vi "Read_capp.vi"(7 "DELAY":u32, 8 "error in (no error)":errorcluster, 9 "String":string, 10 "REFF":refnum<visa-resource-name>, 11 "E4990A":refnum<visa-resource-name>) -> (0 "error out":errorcluster, 1 "Read Buffer":string, 2 "REFFout":refnum<visa-resource-name>, 3 "E4990A out":refnum<visa-resource-name>, 4 "data":dbl)   [LabVIEW 2012]
uses:
  <vilib>/Analysis/baseanly.llb/Mean (DBL).vi
  <vilib>/Analysis/NI_AALBase.lvlib
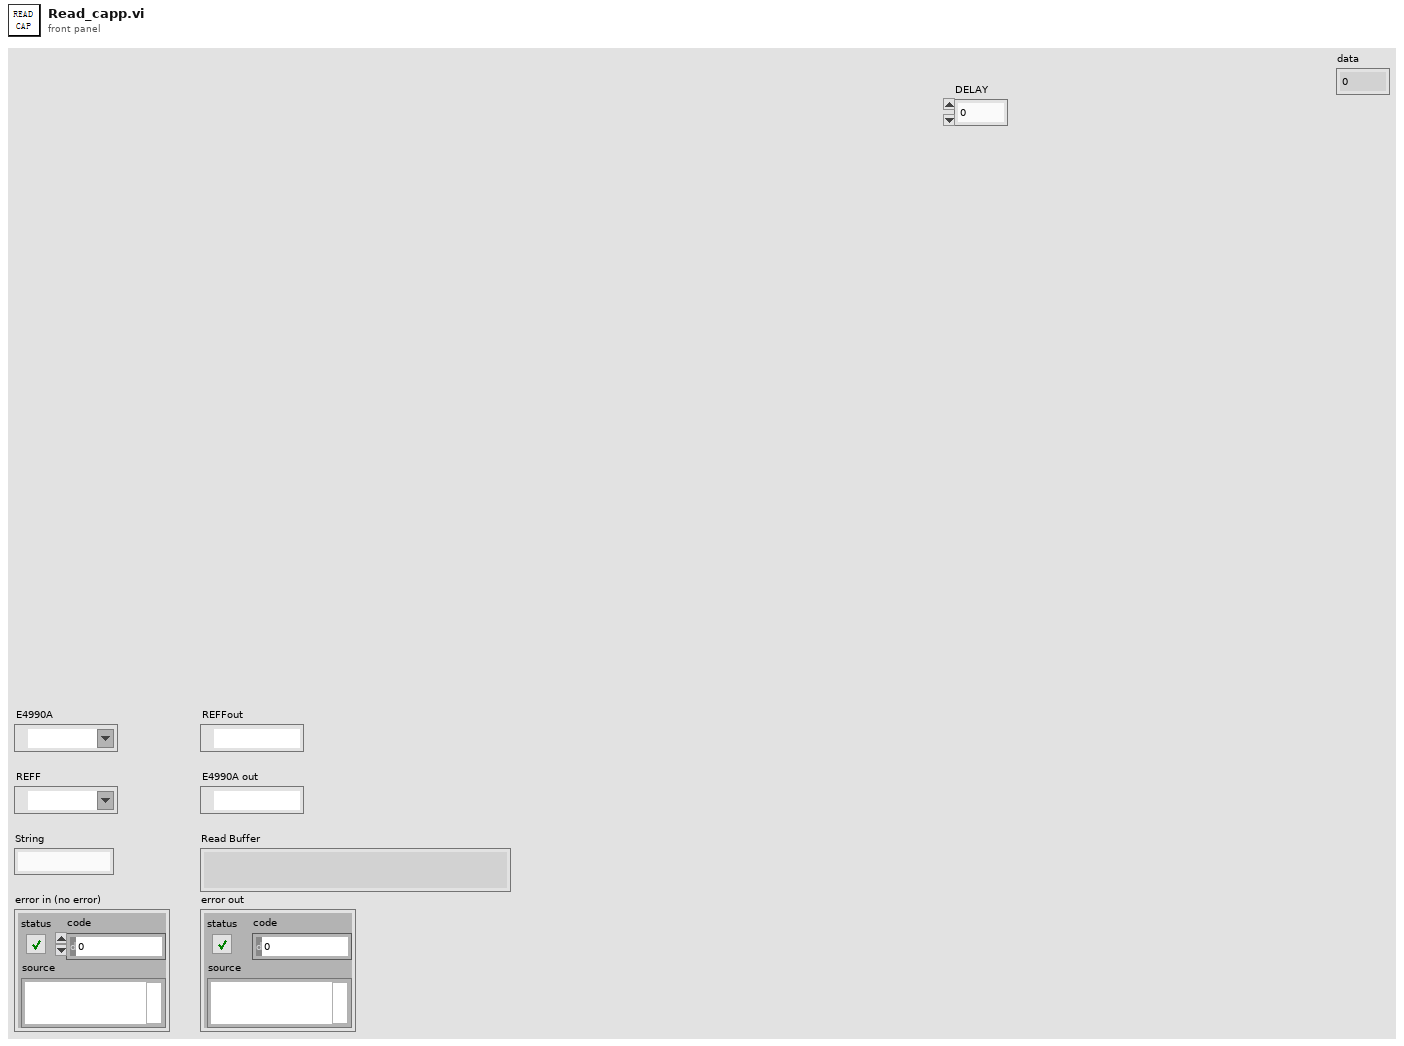
[diagram p1: front panel]
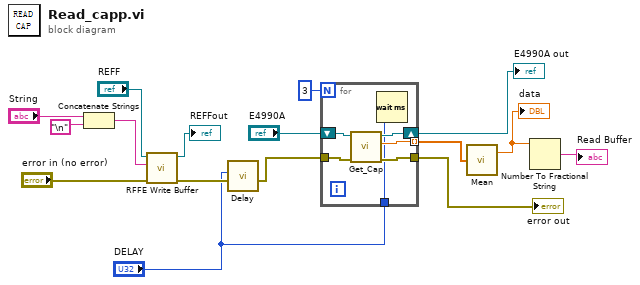
[diagram p0: block diagram]
diagram:
  n1 = Concatenate Strings("String", "\n") -> (w6:string)
  n2 = call "RFFE Write Buffer.vi"("error in (no error)"="error in (no error)", "write buffer"=w6, "VISA resource name"="REFF") -> ("error out"=w14:errorcluster, "VISA resource name out"=→"REFFout":refnum<visa-resource-name>)  [unwired: 7 in]
  n3 = call "Delay.vi"("error in (no error)"=w14, "milliseconds to wait"="DELAY") -> ("error out"=w15:errorcluster)  [unwired: 9 in]
  n4 = for {
    N: 3 -> [_]
    tunnel: [w22] -> w16
    tunnel: w15 -> [w21]
    tunnel: [w18] -> w5 mode=indexing
    shift-right: [w20] -> w13
    shift-left: "E4990A" -> [w19]
    tunnel: "DELAY" -> [w17]
    n5 = call "Get_Cap.vi"("error in (no error)"=w21, "VISA Refnum in"=w19) -> ("error out"=w22:errorcluster, "Numeric"=w18:dbl, "VISA Refnum out"=w20:refnum<visa-resource-name>)  [unwired: 6 in, 1 out]
    n6 = Wait (ms)(milliseconds to wait=w17) -> ()  [unwired: 1 out]
  }
  "error out" <- w16
  "E4990A out" <- w13
  n7 = call-poly <vilib>:"Mean.vi"("X"=w5) -> ("mean"=w4:dbl)  [unwired: 1 out]
  "data" <- w4
  n8 = Number To Fractional String(number=w4) -> (F-format string=→"Read Buffer":string)  [unwired: 3 in]
